vi "SelfTest.vi"(8 "error in (no error)":errorcluster, 11 "CS++DeviceActor in":refnum<class "CS++DeviceActor.lvclass">) -> (0 "error out":errorcluster, 3 "CS++DeviceActor out":refnum<class "CS++DeviceActor.lvclass">)   [LabVIEW 2013, in "CS++DeviceActor.lvlib" / "CS++DeviceActor.lvclass"]
doc: "Perform device selftest."
uses:
  CS++DeviceActor.lvclass
  CS++DeviceActor.lvclass/CS++DeviceActor.ctl
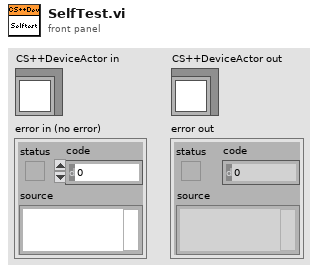
[diagram p1: front panel]
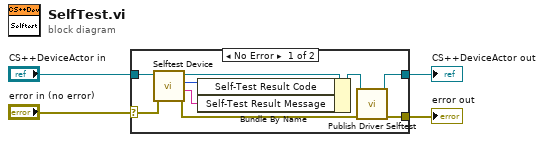
[diagram p0: block diagram]
diagram:
  n1 = case shown="No Error" "error in (no error)" {
    selector: "error in (no error)" -> [w13 w15]
    tunnel: [w7 w15] -> w3
    tunnel: [w5 w14] -> w1
    tunnel: "CS++DeviceActor in" -> [w12 w14]
    frame No Error {
      n2 = call-dynamic "Selftest Device.vi"("error in (no error)"=w13, "CS++DeviceActor in"=w12) -> ("error out"=w8:errorcluster, "Self-Test Result Message"=w9:string, "Self-Test Result Code"=w10:i32, "CS++DeviceActor out"=w11:refnum<class "CS++DeviceActor.lvclass">)  [unwired: 6 in]
      n3 = Bundle By Name(cluster=w11, "Self-Test Result Code"=w10, "Self-Test Result Message"=w9) -> (w6:refnum<class "CS++DeviceActor.lvclass">)
      n4 = call "Publish Driver Selftest.vi"("error in (no error)"=w8, "CS++DeviceActor in"=w6) -> ("error out"=w7:errorcluster, "CS++DeviceActor out"=w5:refnum<class "CS++DeviceActor.lvclass">)  [unwired: 8 in]
    }
    frame Error {
    }
  }
  "error out" <- w3
  "CS++DeviceActor out" <- w1
